vi "Send_sum_wave.vi"(0 "VISA resource name":refnum<visa-resource-name>, 1 "Frequency":dbl, 2 "Phase 1":dbl, 3 "Cant. Freq":dbl, 4 "Phase 2":dbl, 5 "Name":string, 6 "Max sample rate":dbl, 7 "no. periods":i32, 9 "Amp 1":dbl, 12 "error in (no error)":errorcluster, 13 "Amp 2":dbl) -> (14 "VISA resource name out":refnum<visa-resource-name>, 19 "error out":errorcluster)   [LabVIEW 2018]
uses:
  <instrlib>/Tektronix AWG 5000 7000 Series/Tektronix AWG 5000 7000 Series.lvlib
panel:
  out "Waveform Graph":waveform(dbl)(graph)
  out "Samples":i32
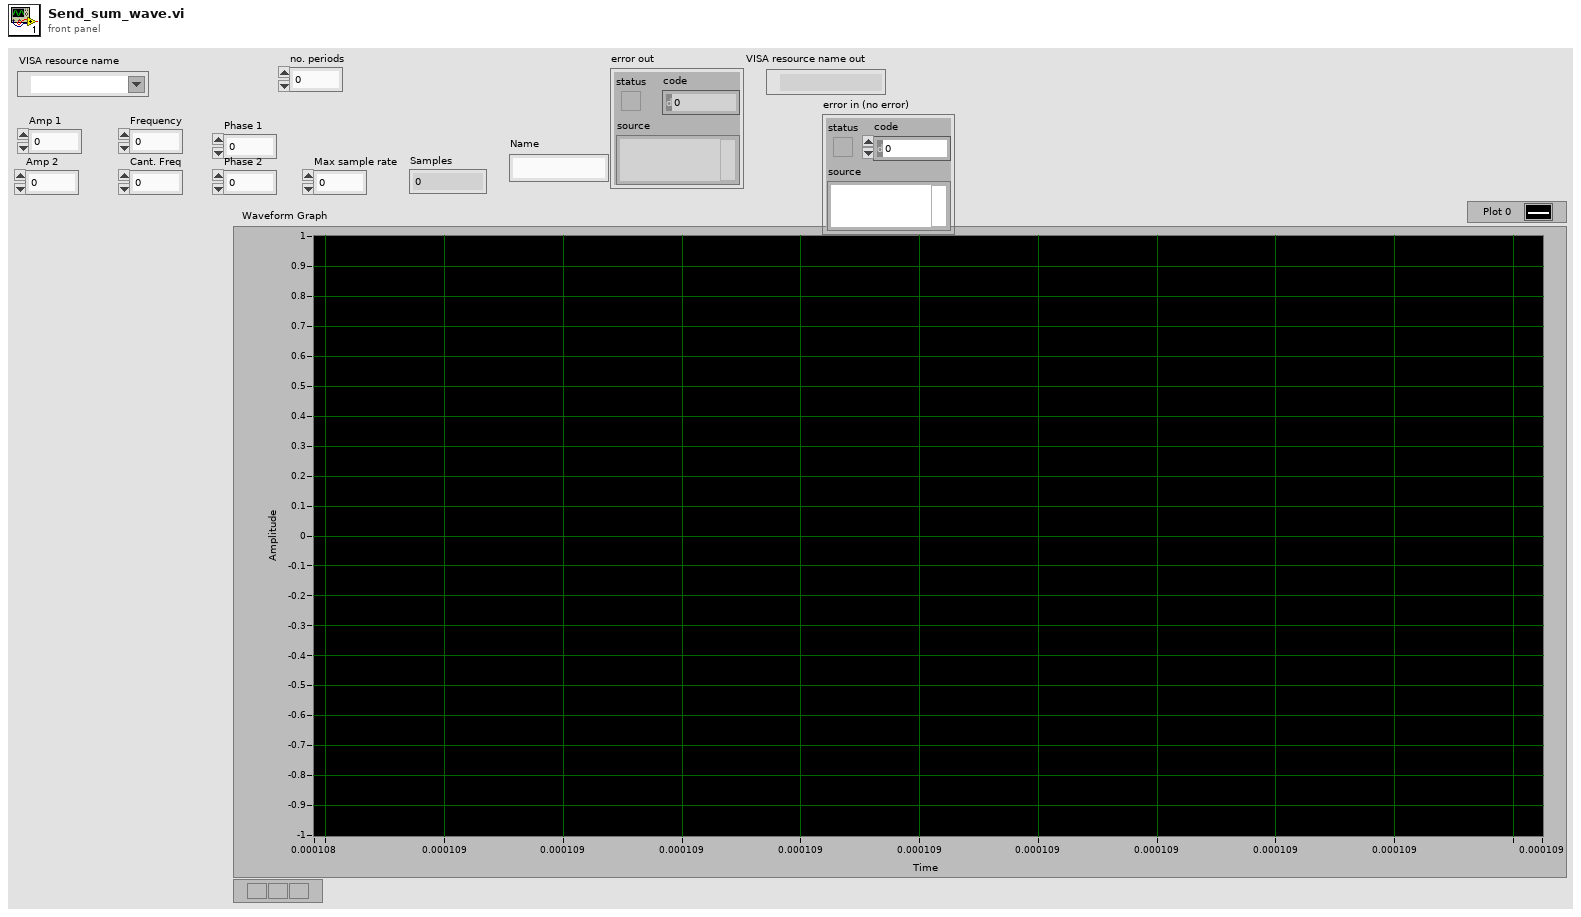
[diagram p1: front panel]
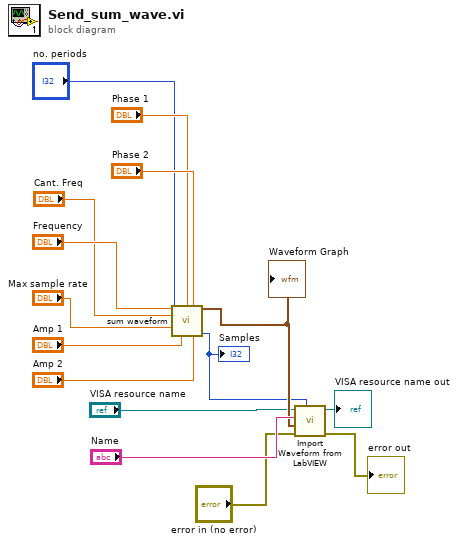
[diagram p0: block diagram]
diagram:
  n1 = call "sum waveform.vi"("RF Freq"="Frequency", "phase 1"="Phase 1", "phase 2"="Phase 2", "Cant. Freq"="Cant. Freq", "no. periods"="no. periods", "Max Sampling Rate"="Max sample rate", "Amp 1 (w0)"="Amp 1", "Amp 2 (w0 + wc)"="Amp 2") -> ("Waveform Graph"=w14:waveform(dbl), "samples"=w8:u32)  [unwired: 6 in]
  "Samples" <- w8
  "Waveform Graph" <- w14
  n2 = call <instrlib>:"Import Waveform from LabVIEW.vi"("Sample Count (1000)"=w8, "error in (no error)"="error in (no error)", "Waveform"=w14, "Waveform Name"="Name", "VISA resource name"="VISA resource name") -> ("error out"=→"error out":errorcluster, "VISA resource name out"=→"VISA resource name out":refnum<visa-resource-name>)  [unwired: 5 in]
